vi "FRCts20_WebMethods_ESP_Comment.vi"(8 "error in (no error)":errorcluster, 9 "Note":T1, 10 "Return Type":T2="mobile", 11 "httpRequestID":u32) -> (0 "error out":errorcluster, 3 "httpRequestID out":u32)   [LabVIEW 2014]
uses:
  Controls/FRCts20_WebMethods_ctl_returntype.ctl
  Backend/source/VI Source/FRCts20_Backend_API/FRCts20_Backend_API_Note.ctl
  Backend/source/VI Source/FRCts20_Backend_API/FRCts20_Backend_API_Request.ctl
  Backend/source/VI Source/FRCts20_Backend_API/FRCts20_Backend_API_Status.ctl
  Backend/source/VI Source/FRCts20_Backend_API/FRCts20_Backend_API_Command_Request.ctl
  Controls/FRCts20_WebMethods_Globals.vi
  Backend/source/VI Source/FRCts20_Backend_API/FRCts20_Backend_API_Request.vi
  <vilib>/wsapi/subVIs/Set String ESP Variable.vi
  <vilib>/wsapi/subVIs/Set Integer ESP Variable.vi
  <vilib>/wsapi/NI_WebServices.lvlib
  FRCts20_WebMethods.lvlib
  Backend/source/VI Source/FRCts20_Backend_API/FRCts20_Backend_API.lvlib
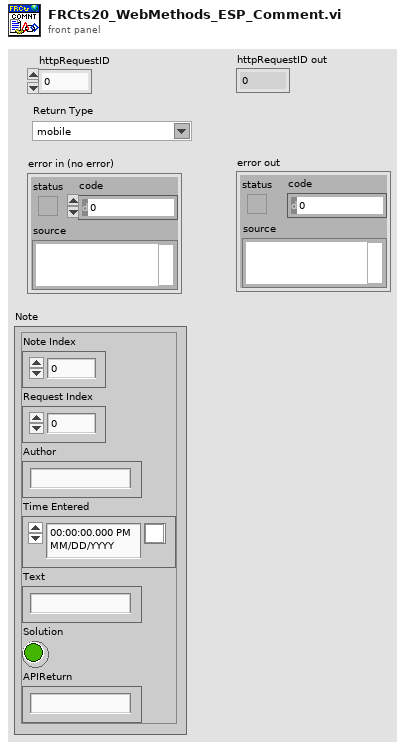
[diagram p1: front panel]
types:
  T1 = typedef "FRCts20_Backend_API.lvlib/FRCts20_Backend_API_Note.ctl" = cluster{"Note Index":u32, "Request Index":u32, "Author":string, "Time Entered":timestamp, "Text":string, "Solution":bool, "APIReturn":string}
  T2 = typedef "FRCts20_WebMethods.lvlib/FRCts20_WebMethods_ctl_returntype.ctl" = string
  T3 = typedef "FRCts20_Backend_API.lvlib/FRCts20_Backend_API_Command_Request.ctl" = string
  T4 = typedef "FRCts20_Backend_API.lvlib/FRCts20_Backend_API_Request.ctl" = cluster{"Request Index":u32, "Description":string, "Status":T5, "Open Date":timestamp, "Last Update":timestamp, "Closed Date":timestamp, "Notes":cluster{"Note Index":u32, "Text":string, "Time Entered":timestamp, "Author":string, "Solution":bool}[], "Team Index":u32, "APIReturn":string}
  T5 = typedef "FRCts20_Backend_API.lvlib/FRCts20_Backend_API_Status.ctl" = enum16{"Open", "In Work", "Closed"}
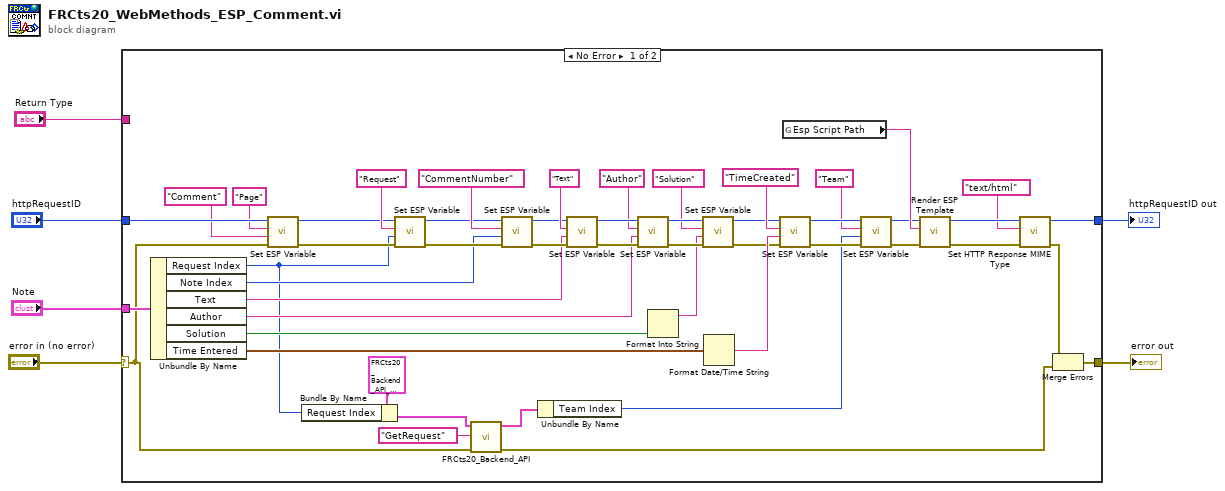
[diagram p0: block diagram]
diagram:
  n1 = case shown="No Error" "error in (no error)" {
    selector: "error in (no error)" -> [w19 w57]
    tunnel: "httpRequestID" -> [w45 w56]
    tunnel: [w53 w56] -> w3
    tunnel: [w9 w57] -> w2
    tunnel: "Return Type" -> [_ _]
    tunnel: "Note" -> [w48 _]
    frame No Error {
      n2 = Unbundle By Name(w48) -> ("Request Index"=w20:u32, "Note Index"=w37:u32, "Text"=w36:string, "Author"=w31:string, "Solution"=w27:bool, "Time Entered"=w35:timestamp)
      n3 = call-poly <vilib>:"Set ESP Variable.vi"("error in (no error)"=w19, "value"="Comment", "key"="Page", "httpRequestID"=w45) -> ("error out"=w22:errorcluster, "httpRequestID out"=w23:u32)  [unwired: 6 in]
      n4 = Bundle By Name(cluster=T4 {"Request Index"=0, "Description"="", "Status"=enum."Open", "Open Date"=timestamp(0 s since 1904-01-01), "Last Update"=timestamp(0 s since 1904-01-01), "Closed Date"=timestamp(0 s since 1904-01-01), "Notes"=[], "Team Index"=0, "APIReturn"=""} ("Request"), "Request Index"=w20) -> (w18:T4)
      n5 = call-poly <vilib>:"Set ESP Variable.vi"("error in (no error)"=w22, "value"=w20, "key"="Request", "httpRequestID"=w23) -> ("error out"=w50:errorcluster, "httpRequestID out"=w49:u32)  [unwired: 6 in]
      n6 = call-poly "FRCts20_Backend_API.vi"("error in (no error)"=w19, "Command"=T3 "GetRequest", "Request In"=w18) -> ("error out"=w7:errorcluster, "Request Out"=w16:T4)  [unwired: 6 in, 1 out]
      n7 = call-poly <vilib>:"Set ESP Variable.vi"("error in (no error)"=w50, "value"=w37, "key"="CommentNumber", "httpRequestID"=w49) -> ("error out"=w39:errorcluster, "httpRequestID out"=w38:u32)  [unwired: 6 in]
      n8 = Unbundle By Name(w16) -> ("Team Index"=w10:u32)
      n9 = call-poly <vilib>:"Set ESP Variable.vi"("error in (no error)"=w39, "value"=w36, "key"="Text", "httpRequestID"=w38) -> ("error out"=w34:errorcluster, "httpRequestID out"=w33:u32)  [unwired: 6 in]
      n10 = call-poly <vilib>:"Set ESP Variable.vi"("error in (no error)"=w34, "value"=w31, "key"="Author", "httpRequestID"=w33) -> ("error out"=w30:errorcluster, "httpRequestID out"=w29:u32)  [unwired: 6 in]
      n11 = Format Into String(w27) -> (resulting string=w26:string)  [unwired: 3 in, 1 out]
      n12 = call-poly <vilib>:"Set ESP Variable.vi"("error in (no error)"=w30, "value"=w26, "key"="Solution", "httpRequestID"=w29) -> ("error out"=w25:errorcluster, "httpRequestID out"=w24:u32)  [unwired: 6 in]
      n13 = Format Date/Time String(seconds (now)=w35) -> (date/time string=w40:string)  [unwired: 2 in]
      n14 = call-poly <vilib>:"Set ESP Variable.vi"("error in (no error)"=w25, "value"=w40, "key"="TimeCreated", "httpRequestID"=w24) -> ("error out"=w13:errorcluster, "httpRequestID out"=w12:u32)  [unwired: 6 in]
      n15 = global read "FRCts20_WebMethods_Globals.vi" "Esp Script Path"() -> (w47:string)
      n16 = call-poly <vilib>:"Set ESP Variable.vi"("error in (no error)"=w13, "value"=w10, "key"="Team", "httpRequestID"=w12) -> ("error out"=w15:errorcluster, "httpRequestID out"=w14:u32)  [unwired: 6 in]
      n17 = call <vilib>:"Render ESP Template.vi"("error in (no error)"=w15, "espName"=w47, "httpRequestID"=w14) -> ("error out"=w54:errorcluster, "httpRequestID out"=w55:u32)  [unwired: 7 in]
      n18 = call <vilib>:"Set HTTP Response MIME Type.vi"("error in (no error)"=w54, "MIME type (text/html)"="text/html", "httpRequestID"=w55) -> ("error out"=w8:errorcluster, "httpRequestID out"=w53:u32)  [unwired: 7 in]
      n19 = Merge Errors(w8, w7) -> (w9:errorcluster)
    }
    frame Error {
    }
  }
  "httpRequestID out" <- w3
  "error out" <- w2
